vi "Boolean_Latch.vi"(5 "Latch Control":bool, 7 "Reset":bool, 9 "Reset on\nFirst Call?(T)":bool=TRUE) -> (8 "Latched?":bool)   [LabVIEW 2015]
doc: "This vi will latch a boolean \"True\" until it is reset with a \"True\" at the Reset input. You have the option to automatically reset the latch on the first call or not. By default, it will reset."
panel:
  # "Boolean Latch - Latches a True value until it is reset.\nCopyright (C) 2002  Edwin Dickens \nedwind@distek.com\n\nThis library is free software; you can redistribute it and/or\nmodify it under the terms of the GNU Lesser General Public\nLicense as published by the Free Software Foundation; either\nversion 2.1 of the License, or (at your option) any later version.\n\nThis library is distributed in the hope that it will be useful, but\nWITHOUT ANY WARRANTY; without even the implied warranty\nof MERCHANTABILITY or FITNESS FOR A PARTICULAR\nPURPOSE. See the GNU Lesser General Public License for\nmore details.\n\nYou should have received a copy of the GNU Lesser General Public\nLicense along with this library; if not, write to the Free Software\nFoundation, Inc., 59 Temple Place,\nSuite 330, Boston, MA 02111-1307 USA"
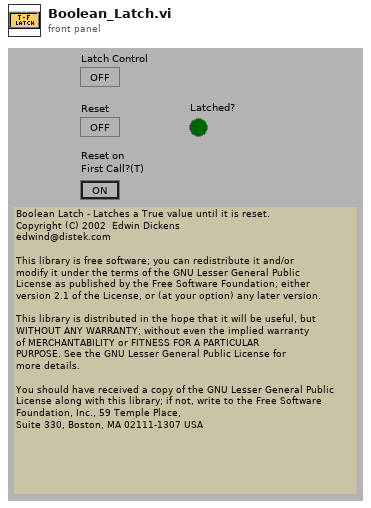
[diagram p1: front panel]
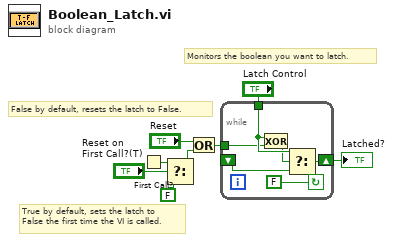
[diagram p0: block diagram]
diagram:
  # "Monitors the boolean you want to latch."
  # "False by default, resets the latch to False."
  # "True by default, sets the latch to\nFalse the first time the VI is called."
  n1 = First Call?() -> (First Call?: T/F=w3:bool)
  n2 = Select(t=w3, s="Reset on\nFirst Call?(T)", f=FALSE) -> (s? t:f=w4:bool)
  n3 = Or(x="Reset", y=w4) -> (x .or. y?=w6:bool)
  n4 = while {
    tunnel: "Latch Control" -> [w14]
    shift-right: [w12] -> w7
    shift-left: _ -> [w11]
    tunnel: w6 -> [w9]
    stop <- FALSE continue-if-true
    n5 = Exclusive Or(1:w9, 2:w14) -> (0:w13:bool)
    n6 = Select(t=w14, s=w13, f=w11) -> (s? t:f=w12:bool)
  }
  "Latched?" <- w7
